vi "TickCountSubtract.vi"(1 "Old Time":u32, 2 "New Time":u32) -> (0 "Time Change":u32)   [LabVIEW 2011, in "UI_Interaction_Manager.lvclass"]
uses:
  UI_Interaction_Manager.lvclass
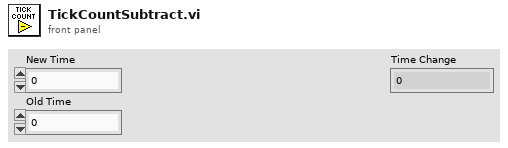
[diagram p1: front panel]
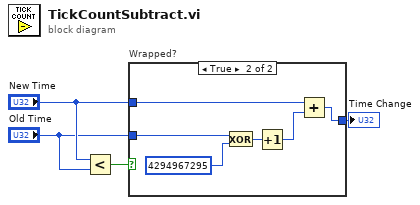
[diagram p0: block diagram]
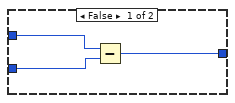
[diagram p2: hidden frame]
diagram:
  n1 = Less?(x="New Time", y="Old Time") -> (x < y?=w4:bool)
  n2 = case "Wrapped?" shown="True" w4 {
    tunnel: "New Time" -> [w7 w10]
    tunnel: "Old Time" -> [w6 w11]
    tunnel: [w5 w8] -> w1
    frame False {
      n3 = Subtract(x=w7, y=w6) -> (x-y=w5:u32)
    }
    frame True {
      n4 = Exclusive Or(1:u32 4294967295 ("y"), 2:w11) -> (0:w13:u32)
      n5 = Increment(x=w13) -> (x+1=w9:u32)
      n6 = Add(x=w10, y=w9) -> (x+y=w8:u32)
    }
  }
  "Time Change" <- w1
